vi "Transcriptor LabVIEW to C code Step 1 and 2 Wires Declarations and Assignements.vi"(8 "error in":errorcluster, 11 "Diagram in":refnum<vi>) -> (2 "wires declarations":string[](array[string]), 3 "end loop refs.":string[](array[string]))   [LabVIEW 2014]
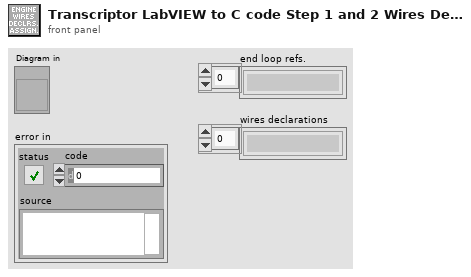
[diagram p1: front panel]
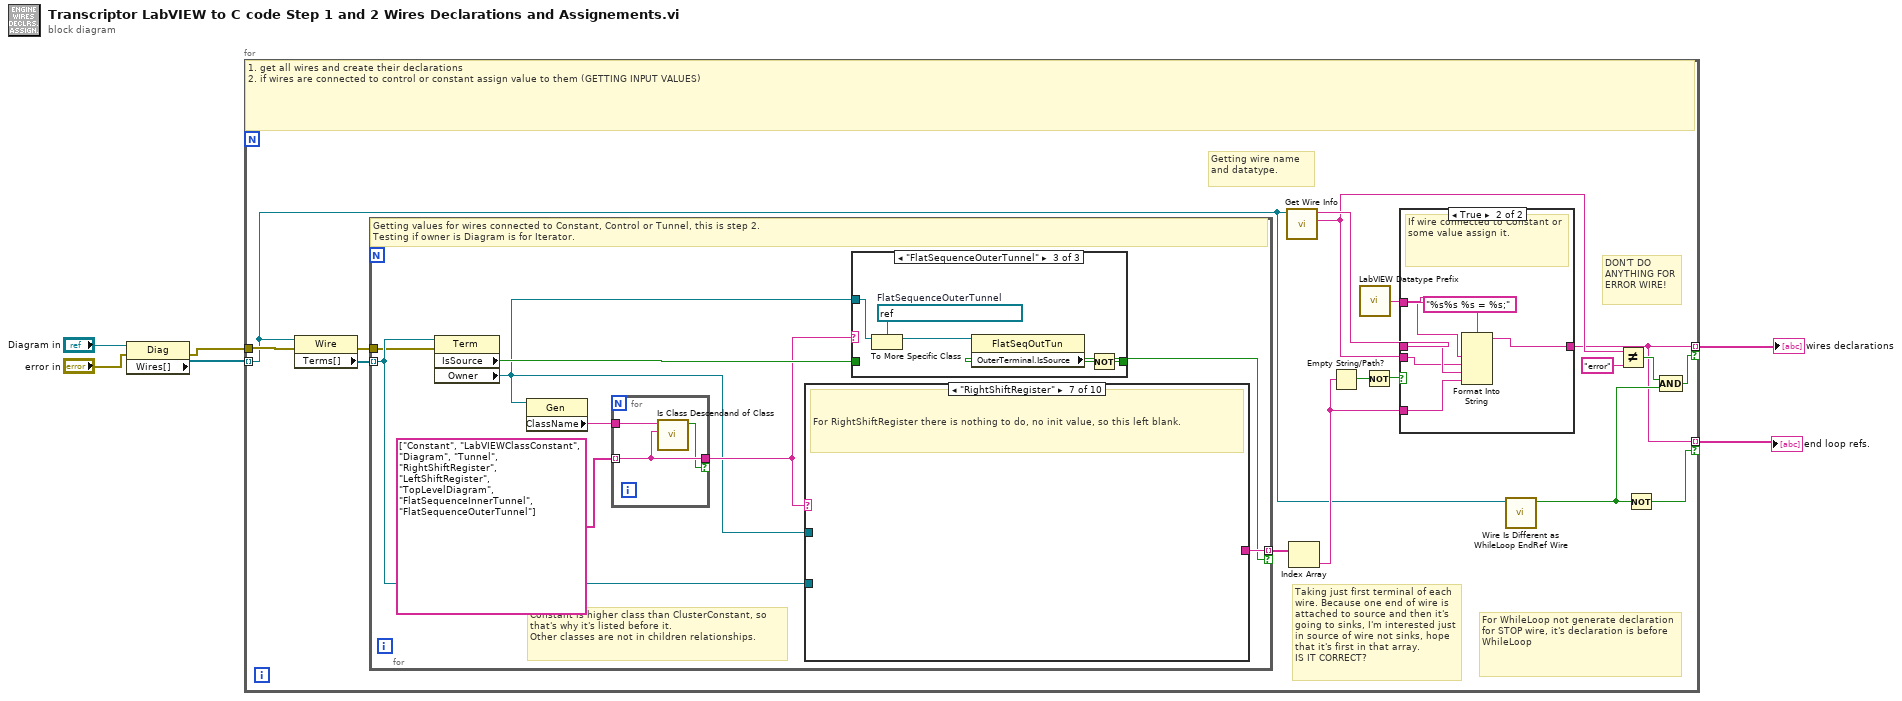
[diagram p0: block diagram]
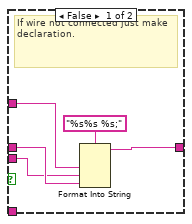
[diagram p2: hidden frame]
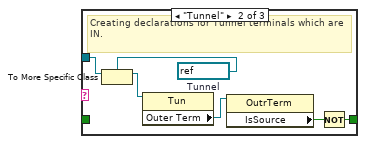
[diagram p4: hidden frame]
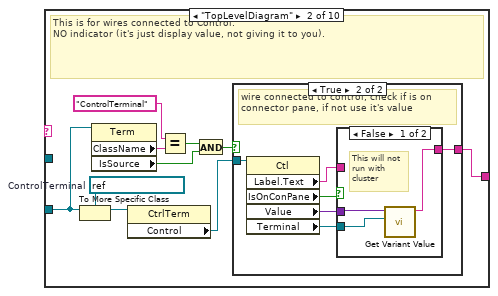
[diagram p6: hidden frame]
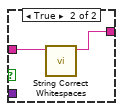
[diagram p8: hidden frame]
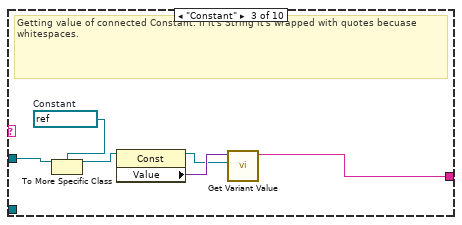
[diagram p9: hidden frame]
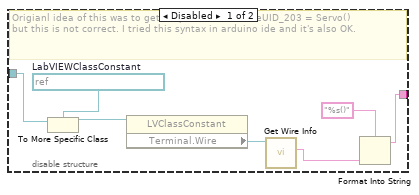
[diagram p11: hidden frame]
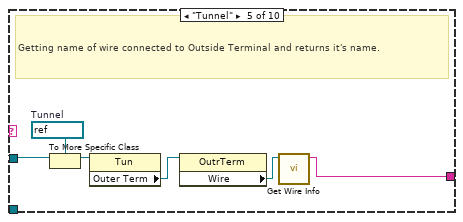
[diagram p12: hidden frame]
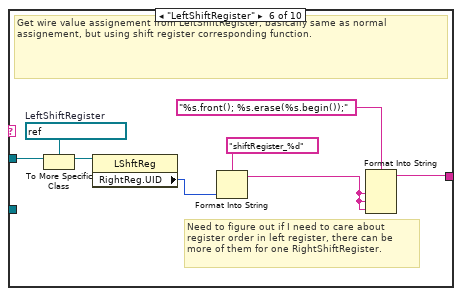
[diagram p13: hidden frame]
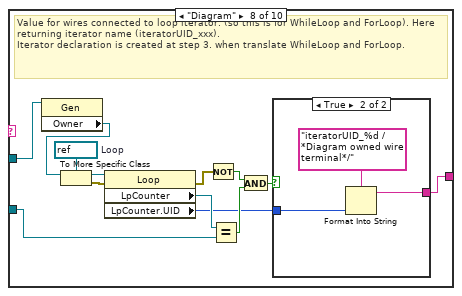
[diagram p14: hidden frame]
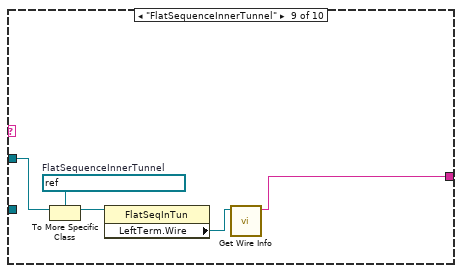
[diagram p16: hidden frame]
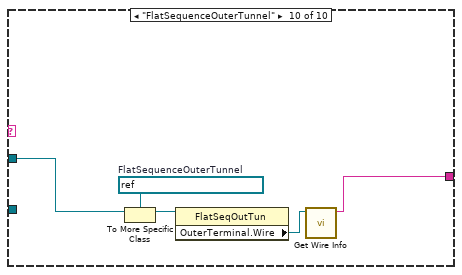
[diagram p17: hidden frame]
diagram:
  n1 = property class="Diag"(reference="Diagram in", error in="error in") -> (error out=w2:errorcluster, "Wires[]"=w1:refnum<vi>[])  [unwired: 1 out]
  n2 = for {
    tunnel: w1 -> [w10] mode=indexing
    tunnel: [w8] -> w6 mode=indexing if=w11
    tunnel: w2 -> [w16]
    tunnel: [w8] -> w5 mode=indexing if=w7
    # "Getting wire name and datatype."
    # "For WhileLoop not generate declaration for STOP wire, it's declaration is before WhileLoop"
    # "Taking just first terminal of each wire. Because one end of wire is attached to source and then it's going to sinks, I'm interested just in source of wire not sinks, hope that it's first in that array.\nIS IT CORRECT?"
    # "DON'T DO ANYTHING FOR ERROR WIRE!"
    # "1. get all wires and create their declarations\n2. if wires are connected to control or constant assign value to them (GETTING INPUT VALUES)"
    n3 = property class="Wire"(reference=w10, error in=w16) -> (error out=w15:errorcluster, "Terms[]"=w23:refnum<vi>[])  [unwired: 1 out]
    n4 = for {
      tunnel: w23 -> [w42] mode=indexing
      tunnel: [w43] -> w22 mode=indexing if=w40
      tunnel: w15 -> [w41]
      # "Constant is higher class than ClusterConstant, so that's why it's listed before it.\nOther classes are not in children relationships."
      # "Getting values for wires connected to Constant, Control or Tunnel, this is step 2.\nTesting if owner is Diagram is for Iterator."
      n5 = property class="Term"(reference=w42, error in=w41) -> ("IsSource"=w39:bool, "Owner"=w35:refnum<vi>)  [unwired: 2 out]
      n6 = property class="Gen"(reference=w35) -> ("ClassName"=w37:string)  [unwired: 1 in, 2 out]
      n7 = for {
        tunnel: string[] ["Constant", "LabVIEWClassConstant", "Diagram", "Tunnel", "RightShiftRegister", "LeftShiftRegister", "TopLevelDiagram", "FlatSequenceInnerTunnel", "FlatSequenceOuterTunnel"] -> [w45] mode=indexing
        tunnel: w37 -> [w46]
        tunnel: [w45] -> w36 if=w44
        n8 = call "Is Class Descendand of Class.vi"("Parent ClassName"=w45, "ClassName"=w46) -> ("is Class descendant?"=w44:bool)  [unwired: 8 in, 1 out]
      }
      n9 = case shown="\"RightShiftRegister\"" w36 {
        tunnel: w35 -> [_ _ w85 w87 w99 w106 _ w121 w125 w130]
        tunnel: [_ w66 w82 w86 w95 w101 _ w111 w126 w132] -> w43
        tunnel: w42 -> [_ w64 _ _ _ _ _ w117 _ _]
        frame Default {
          # "If wire is not wired to anything from what I have to read value, output is default Variant value (hope that is empty Variant), and there will be just wire declaration without assignement in generated code."
        }
        frame "TopLevelDiagram" {
          w68 = refnum<vi> refnum  # ControlTerminal
          # "This is for wires connected to Control.\nNO indicator (it's just display value, not giving it to you)."
          n10 = To More Specific Class(target class=w68, reference=w64) -> (specific class reference=w67:refnum<vi>)  [unwired: 1 in, 1 out]
          n11 = property class="Term"(reference=w64) -> ("ClassName"=w63:string, "IsSource"=w59:bool)  [unwired: 1 in, 2 out]
          n12 = property class="CtrlTerm"(reference=w67) -> ("Control"=w62:refnum<vi>)  [unwired: 1 in, 2 out]
          n13 = Equal?(x="ControlTerminal", y=w63) -> (x = y?=w60:bool)
          n14 = And(x=w60, y=w59) -> (x .and. y?=w61:bool)
          n15 = case shown="True" w61 {
            tunnel: [_ w72] -> w66
            tunnel: w62 -> [_ w74]
            frame False {
              # "wire connected to indicator, do nothing"
            }
            frame True {
              # "wire connected to control, check if is on connector pane, if not use it's value"
              n16 = property class="Ctl"(reference=w74) -> ("Label.Text"=w73:string, "IsOnConPane"=w71:bool, "Value"=w70:variant, "Terminal"=w69:refnum<vi>)  [unwired: 1 in, 2 out]
              n17 = case shown="False" w71 {
                tunnel: w73 -> [_ w79]
                tunnel: [w76 w78] -> w72
                tunnel: w70 -> [w77 _]
                tunnel: w69 -> [w75 _]
                frame False {
                  # "This will not\nrun with\ncluster"
                  n18 = call "Get Variant Value.vi"("GObj Refnum"=w75, "Variant in"=w77) -> ("Variant value as string"=w76:string)  [unwired: 9 in]
                }
                frame True {
                  n19 = call "String Correct Whitespaces.vi"("String in"=w79) -> ("String out"=w78:string)  [unwired: 10 in]
                }
              }
            }
          }
        }
        frame "Constant" {
          w84 = refnum<vi> refnum  # Constant
          # "Getting value of connected Constant. If it's String it's wrapped with quotes becuase whitespaces."
          n20 = To More Specific Class(target class=w84, reference=w85) -> (specific class reference=w83:refnum<vi>)  [unwired: 1 in, 1 out]
          n21 = property class="Const"(reference=w83) -> (reference out=w80:refnum<vi>, "Value"=w81:variant)  [unwired: 1 in, 1 out]
          n22 = call "Get Variant Value.vi"("GObj Refnum"=w80, "Variant in"=w81) -> ("Variant value as string"=w82:string)  [unwired: 9 in]
        }
        frame "LabVIEWClassConstant" {
          # "For class constant connected to wire there is nothing to get, we have to in the end obtain just normal C++ object declaration ie. for Servo class:\nServo wireUID_203;"
          n23 = disable-structure shown="Enabled" {
            disable-tunnel: w87 -> [w94 _]
            disable-tunnel: [w89 _] -> w86
            frame Disabled {
              w93 = refnum<vi> refnum  # LabVIEWClassConstant
              # "Origianl idea of this was to get output as Servo wireUID_203 = Servo()\nbut this is not correct. I tried this syntax in arduino ide and it's also OK."
              n24 = To More Specific Class(target class=w93, reference=w94) -> (specific class reference=w92:refnum<vi>)  [unwired: 1 in, 1 out]
              n25 = property class="LVClassConstant"(reference=w92) -> ("Terminal.Wire"=w91:refnum<vi>)  [unwired: 1 in, 2 out]
              n26 = call "Get Wire Info.vi"("Wire"=w91) -> ("wire datatype"=w88:string)  [unwired: 9 in, 1 out]
              n27 = Format Into String(format string="%s()", w88) -> (resulting string=w89:string)  [unwired: 2 in, 1 out]
            }
            frame Enabled {
              # "Nothing to return, so in the end object wire declaration is without initilization (we are working normal memory of MCU NOT in stack!)"
            }
          }
        }
        frame "Tunnel" {
          w100 = refnum<vi> refnum  # Tunnel
          # "Getting name of wire connected to Outside Terminal and returns it's name."
          n28 = To More Specific Class(target class=w100, reference=w99) -> (specific class reference=w98:refnum<vi>)  [unwired: 1 in, 1 out]
          n29 = property class="Tun"(reference=w98) -> ("Outer Term"=w97:refnum<vi>)  [unwired: 1 in, 2 out]
          n30 = property class="OutrTerm"(reference=w97) -> ("Wire"=w96:refnum<vi>)  [unwired: 1 in, 2 out]
          n31 = call "Get Wire Info.vi"("Wire"=w96) -> ("wire label"=w95:string)  [unwired: 9 in, 1 out]
        }
        frame "LeftShiftRegister" {
          w108 = refnum<vi> refnum  # LeftShiftRegister
          # "Need to figure out if I need to care about register order in left register, there can be more of them for one RightShiftRegister."
          # "Get wire value assignement from LeftShiftRegister, basically same as normal assignement, but using shift register corresponding function."
          n32 = To More Specific Class(target class=w108, reference=w106) -> (specific class reference=w107:refnum<vi>)  [unwired: 1 in, 1 out]
          n33 = property class="LShftReg"(reference=w107) -> ("RightReg.UID"=w104:i32)  [unwired: 1 in, 2 out]
          n34 = Format Into String(format string="shiftRegister_%d", w104) -> (resulting string=w102:string)  [unwired: 2 in, 1 out]
          n35 = Format Into String(format string="%s.front(); %s.erase(%s.begin());", w102, w102, w102) -> (resulting string=w101:string)  [unwired: 2 in, 1 out]
        }
        frame "RightShiftRegister" {
          # "For RightShiftRegister there is nothing to do, no init value, so this left blank."
        }
        frame "Diagram" {
          w120 = refnum<vi> refnum  # Loop
          # "Value for wires connected to loop iterator. (so this is for WhileLoop and ForLoop). Here returning iterator name (iteratorUID_xxx).\nIterator declaration is created at step 3. when translate WhileLoop and ForLoop."
          n36 = property class="Gen"(reference=w121) -> ("Owner"=w109:refnum<vi>)  [unwired: 1 in, 2 out]
          n37 = To More Specific Class(target class=w120, reference=w109) -> (specific class reference=w119:refnum<vi>, error out=w116:errorcluster)  [unwired: 1 in]
          n38 = property class="Loop"(reference=w119, error in=w116) -> (error out=w115:errorcluster, "LpCounter"=w118:refnum<vi>, "LpCounter.UID"=w110:i32)  [unwired: 1 out]
          n39 = Not(x=w115) -> (.not. x?=w114:bool)
          n40 = Equal?(x=w118, y=w117) -> (x = y?=w113:bool)
          n41 = And(x=w114, y=w113) -> (x .and. y?=w112:bool)
          n42 = case shown="True" w112 {
            tunnel: [_ w124] -> w111
            tunnel: w110 -> [_ w122]
            frame False {
            }
            frame True {
              n43 = Format Into String(format string="iteratorUID_%d /*Diagram owned wire terminal*/", w122) -> (resulting string=w124:string)  [unwired: 2 in, 1 out]
            }
          }
        }
        frame "FlatSequenceInnerTunnel" {
          w129 = refnum<vi> refnum  # FlatSequenceInnerTunnel
          n44 = To More Specific Class(target class=w129, reference=w125) -> (specific class reference=w128:refnum<vi>)  [unwired: 1 in, 1 out]
          n45 = property class="FlatSeqInTun"(reference=w128) -> ("LeftTerm.Wire"=w127:refnum<vi>)  [unwired: 1 in, 2 out]
          n46 = call "Get Wire Info.vi"("Wire"=w127) -> ("wire label"=w126:string)  [unwired: 9 in, 1 out]
        }
        frame "FlatSequenceOuterTunnel" {
          w134 = refnum<vi> refnum  # FlatSequenceOuterTunnel
          n47 = To More Specific Class(target class=w134, reference=w130) -> (specific class reference=w133:refnum<vi>)  [unwired: 1 in, 1 out]
          n48 = property class="FlatSeqOutTun"(reference=w133) -> ("OuterTerminal.Wire"=w131:refnum<vi>)  [unwired: 1 in, 2 out]
          n49 = call "Get Wire Info.vi"("Wire"=w131) -> ("wire label"=w132:string)  [unwired: 9 in, 1 out]
        }
      }
      n50 = case shown="\"FlatSequenceOuterTunnel\"" w36 {
        tunnel: [w47 w48 w55] -> w40
        tunnel: w39 -> [w47 _ _]
        tunnel: w35 -> [_ w50 w56]
        frame Default {
          # "For all others Terminal.Owner don't need to do anything else."
        }
        frame "Tunnel" {
          w52 = refnum<vi> refnum  # Tunnel
          # "Creating declarations for Tunnel terminals which are IN."
          n51 = To More Specific Class(target class=w52, reference=w50) -> (specific class reference=w53:refnum<vi>)  [unwired: 1 in, 1 out]
          n52 = property class="Tun"(reference=w53) -> ("Outer Term"=w51:refnum<vi>)  [unwired: 1 in, 2 out]
          n53 = property class="OutrTerm"(reference=w51) -> ("IsSource"=w49:bool)  [unwired: 1 in, 2 out]
          n54 = Not(x=w49) -> (.not. x?=w48:bool)
        }
        frame "FlatSequenceOuterTunnel" {
          w57 = refnum<vi> refnum  # FlatSequenceOuterTunnel
          n55 = To More Specific Class(target class=w57, reference=w56) -> (specific class reference=w58:refnum<vi>)  [unwired: 1 in, 1 out]
          n56 = property class="FlatSeqOutTun"(reference=w58) -> ("OuterTerminal.IsSource"=w54:bool)  [unwired: 1 in, 2 out]
          n57 = Not(x=w54) -> (.not. x?=w55:bool)
        }
      }
    }
    n58 = call "Get Wire Info.vi"("Wire"=w10) -> ("wire datatype"=w19:string, "wire label"=w20:string)  [unwired: 9 in]
    n59 = Index Array(array=w22) -> (element=w13:string)  [unwired: 1 in]
    n60 = Empty String/Path?(string/path=w13) -> (empty?=w21:bool)
    n61 = call "LabVIEW Datatype Prefix.vi"() -> ("datatype prefix"=w14:string)
    n62 = Not(x=w21) -> (.not. x?=w17:bool)
    n63 = case shown="True" w17 {
      tunnel: w20 -> [w26 w31]
      tunnel: w19 -> [w25 w30]
      tunnel: w13 -> [_ w33]
      tunnel: [w27 w32] -> w8
      tunnel: w14 -> [w24 w29]
      frame False {
        # "If wire not connected just make declaration."
        n64 = Format Into String(format string="%s%s %s;", w24, w25, w26) -> (resulting string=w27:string)  [unwired: 2 in, 1 out]
      }
      frame True {
        # "If wire connected to Constant or some value assign it."
        n65 = Format Into String(format string="%s%s %s = %s;", w29, w30, w31, w33) -> (resulting string=w32:string)  [unwired: 2 in, 1 out]
      }
    }
    n66 = call "Wire Is Different as WhileLoop EndRef Wire.vi"("Wire in"=w10) -> ("is different than WhileLoop endref?"=w9:bool)  [unwired: 10 in]
    n67 = Not Equal?(x=w19, y="error") -> (x != y?=w12:bool)
    n68 = Not(x=w9) -> (.not. x?=w7:bool)
    n69 = Compound Arithmetic op=AND(w12, w9) -> (w11:bool)
  }
  "wires declarations" <- w6
  "end loop refs." <- w5
